vi "niDTS WLAN INSTR RX Configure.vi"(4 "MAC Address":string="FF:FF:FF:FF:FF:FF", 6 "Port Names":string[](array[string])=["RF0/Port0", "RF1/Port1", "RF0/Port6", "RF1/Port7"], 8 "error in (no error)":errorcluster, 9 "Payload length limit":i32=12000, 10 "Channel Secondary Factor":enum16{"-1", "1", "0"}(ring)=enum."1", 11 "niDTS WLAN INSTR RX in":refnum<class "niDTS WLAN INSTR RX.lvclass">) -> (0 "error out":errorcluster, 3 "niDTS WLAN INSTR RX out":refnum<class "niDTS WLAN INSTR RX.lvclass">)   [LabVIEW 2015, in "niDTS WLAN.lvlib" / "niDTS WLAN INSTR RX.lvclass"]
uses:
  niDTS WLAN INSTR RX.lvclass
  niDTS WLAN INSTR RX.lvclass/niDTS WLAN INSTR RX.ctl
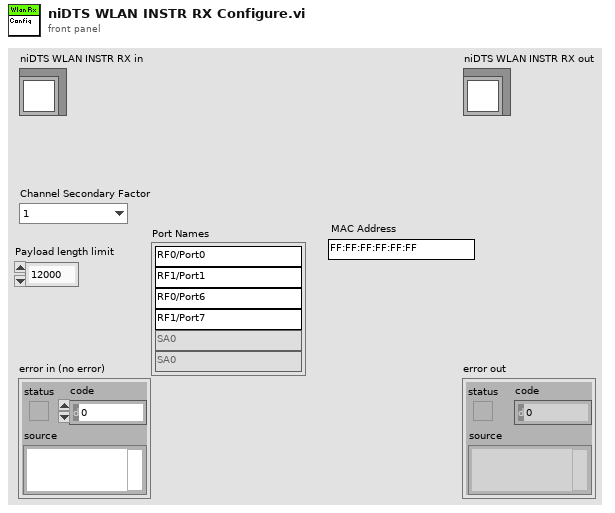
[diagram p1: front panel]
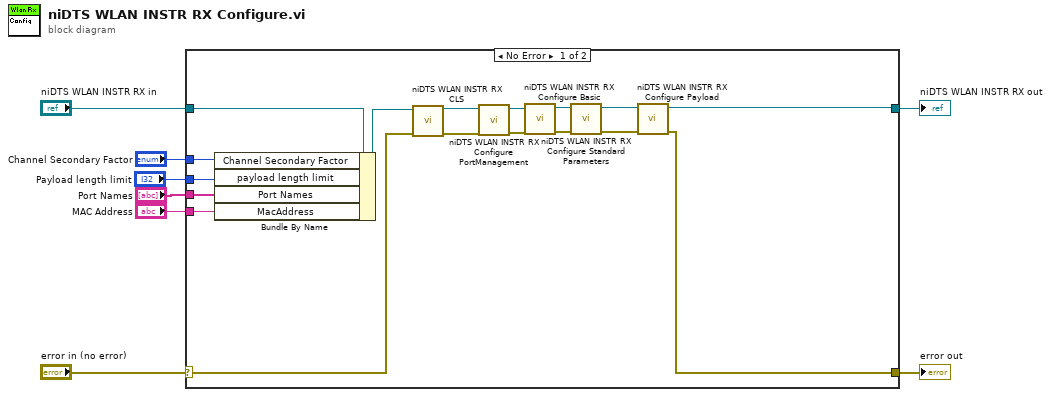
[diagram p0: block diagram]
diagram:
  n1 = case shown="No Error" "error in (no error)" {
    selector: "error in (no error)" -> [w11 w27]
    tunnel: [w17 w27] -> w7
    tunnel: [w19 w26] -> w5
    tunnel: "niDTS WLAN INSTR RX in" -> [w22 w26]
    tunnel: "Channel Secondary Factor" -> [w20 _]
    tunnel: "Payload length limit" -> [w21 _]
    tunnel: "Port Names" -> [w16 _]
    tunnel: "MAC Address" -> [w13 _]
    frame No Error {
      n2 = Bundle By Name(cluster=w22, "Channel Secondary Factor"=w20, "payload length limit"=w21, "Port Names"=w16, "MacAddress"=w13) -> (w12:refnum<class "niDTS WLAN INSTR RX.lvclass">)
      n3 = call-dynamic "niDTS WLAN INSTR RX CLS.vi"("error in (no error)"=w11, "niDTS WLAN INSTR RX in"=w12) -> ("error out"=w10:errorcluster, "niDTS WLAN INSTR RX out"=w9:refnum<class "niDTS WLAN INSTR RX.lvclass">)  [unwired: 8 in]
      n4 = call-dynamic "niDTS WLAN INSTR RX Configure PortManagement.vi"("error in (no error)"=w10, "niDTS WLAN INSTR RX in"=w9) -> ("error out"=w14:errorcluster, "niDTS WLAN INSTR RX out"=w15:refnum<class "niDTS WLAN INSTR RX.lvclass">)  [unwired: 8 in]
      n5 = call-dynamic "niDTS WLAN INSTR RX Configure Basic.vi"("error in (no error)"=w14, "niDTS WLAN INSTR RX in"=w15) -> ("error out"=w23:errorcluster, "niDTS WLAN INSTR RX out"=w25:refnum<class "niDTS WLAN INSTR RX.lvclass">)  [unwired: 8 in]
      n6 = call-dynamic "niDTS WLAN INSTR RX Configure Standard Parameters.vi"("error in (no error)"=w23, "niDTS WLAN INSTR RX in"=w25) -> ("error out"=w18:errorcluster, "niDTS WLAN INSTR RX out"=w24:refnum<class "niDTS WLAN INSTR RX.lvclass">)  [unwired: 8 in]
      n7 = call-dynamic "niDTS WLAN INSTR RX Configure Payload.vi"("error in (no error)"=w18, "niDTS WLAN INSTR RX in"=w24) -> ("error out"=w17:errorcluster, "niDTS WLAN INSTR RX out"=w19:refnum<class "niDTS WLAN INSTR RX.lvclass">)  [unwired: 8 in]
    }
    frame Error {
    }
  }
  "error out" <- w7
  "niDTS WLAN INSTR RX out" <- w5
